vi "8,5-Test of Comm Protocol.vi"() -> ()   [LabVIEW 2010]
uses:
  2-Low Neurons/2.2-Where Control.ctl
  2-Low Neurons/2.2-Where Indicator.ctl
panel:
  out "Observed Command on Device":u8[](array[numeric])
  in  "Prepared Command to Device":u8[](array[numeric])
  out "Observed Reply from Device":u8[](array[numeric])
  in  "Prepared Reply on Device":u8[](array[numeric])
  in  "stop":bool
  out "2.2 Where Indicator":T1
  in  "2.2 Where Control":T2
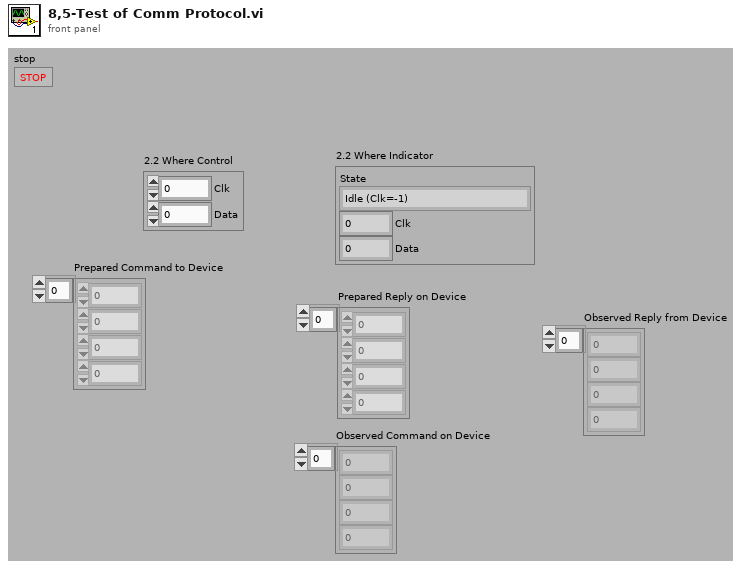
[diagram p1: front panel]
types:
  T1 = typedef "2.2-Where Indicator.ctl" = cluster{"State":enum8{"Idle (Clk=-1)", "Sending(Clk*==Clk+1?Clk=Clk*:;)", "Receiving(Clk*==Clk?Clk++:;)"}, "Clk":i8, "Data":u8}
  T2 = typedef "2.2-Where Control.ctl" = cluster{"Clk":i8, "Data":u8}
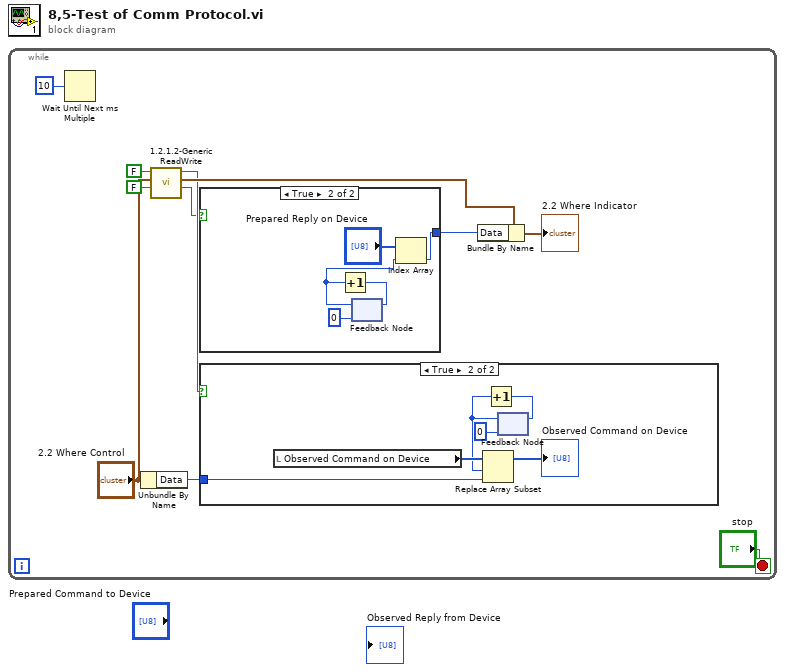
[diagram p0: block diagram]
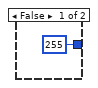
[diagram p2: hidden frame]
diagram:
  n1 = while {
    stop <- "stop" stop-if-true
    n2 = Wait Until Next ms Multiple(millisecond multiple=u32 10) -> ()  [unwired: 1 out]
    n3 = Unbundle By Name("2.2 Where Control") -> ("Data"=w3:u8)
    n4 = call "1.2.1.2-Generic ReadWrite.vi"("RS232-1\\Port1 Read Timeout"=FALSE ("RS232-1\\Port1 Read Timeout"), "2.2 Where Control"="2.2 Where Control", "RS232-1\\Port1 Write Timeout"=FALSE ("RS232-1\\Port1 Write Timeout")) -> ("RS232-1\\Port1 Read Case"=w6:bool, "2.2 Where Indicator"=w10:T1, "RS232-1\\Port1 Write Case"=w7:bool)  [unwired: 2 in]
    n5 = case shown="True" w6 {
      tunnel: [u8 255 ("Numeric") w13] -> w5
      frame False {
      }
      frame True {
        n6 = feedback #1(0) -> (w16:i32)
        n7 = Increment(x=w16) -> (x+1=w15:i32)
        n8 = feedback-in #1(w15) -> ()
        n9 = Index Array(array="Prepared Reply on Device", index=w16) -> (element=w13:u8)
      }
    }
    n10 = case shown="True" w7 {
      tunnel: w3 -> [_ w18]
      frame False {
      }
      frame True {
        n11 = local read "Observed Command on Device"() -> (w23:u8[])
        n12 = feedback #2(0) -> (w19:i32)
        n13 = Replace Array Subset(array=w23, new element=w18, index=w19) -> (→"Observed Command on Device":u8[])
        n14 = Increment(x=w19) -> (x+1=w20:i32)
        n15 = feedback-in #2(w20) -> ()
      }
    }
    n16 = Bundle By Name(cluster=w10, "Data"=w5) -> (→"2.2 Where Indicator":T1)
  }
